vi "Auto Intake Mode.vi"(7 "Intake Current Angle":dbl, 10 "Ball Loaded?":bool) -> (1 "Target Height":dbl, 2 "Roller Speed":dbl, 3 "Angle Power":dbl)   [LabVIEW 2015]
uses:
  Common Code/Intake Commands.ctl
  Robot Global Data.vi
  <vilib>/addons/control/pid/pid.llb/PID (DBL).vi
  <vilib>/addons/control/pid/NI_PID_pid.lvlib
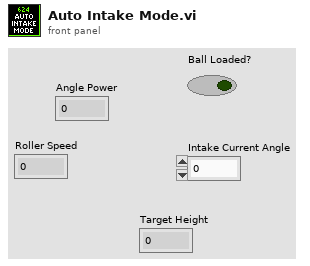
[diagram p1: front panel]
types:
  T1 = typedef "Intake Commands.ctl" = enum16{"Unload", "Load", "Drop low", "Idle"}
  T2 = typedef "Dashboard Control Data.ctl" = cluster{"Encoder Control":T3, "Steer PID output":cluster{"output high":dbl, "output low":dbl}, " Steer PID gains":cluster{"proportional gain (Kc)":dbl, "integral time (Ti, min)":dbl, "derivative time (Td, min)":dbl}, "Drivetrain Settings":T4, "Vision Packet":T5, "Dashboard Drivetrain Command":T6, "Info/Command Cluster":T8, "Ball Vision Packet":T9, "Intake Presets":T11, "Intake Encoder Control":T13, "Climb Presets":T14, "Goal Output Range":cluster{"output high":dbl, "output low":dbl}, "Enabled Systems":T15, "Auton Presets":T16, "Pressure M":dbl, "Pressure B":dbl, "Vision Timeout":dbl, "Auto-Shift":T17, "Catapult Setpoints":T18}
  T3 = typedef "Encoder Control.ctl" = cluster{"Right Tick Constant":dbl, "Left Tick Constant":dbl, "Reset?":bool, "Y Dist":cluster{"PID gains":cluster{"proportional gain (Kc)":dbl, "integral time (Ti, min)":dbl, "derivative time (Td, min)":dbl}}, "Y Stop Thresh":dbl, "Y Stop Speed":dbl}
  T4 = typedef "Drivetrain Settings.ctl" = cluster{"Gyro Tolerance":dbl, "Throttle Ramp (ms)":dbl, "Kv":dbl, "Ka":dbl, "Feed Forward P":dbl, "Feed Forward D":dbl, "Goal Vision PID gains":cluster{"proportional gain (Kc)":dbl, "integral time (Ti, min)":dbl, "derivative time (Td, min)":dbl}, "Goal Detection Window":dbl, "Creep Rate":dbl, "Vision Throttle Threshold":dbl, "Min Turn Output":dbl, "Left Batter Angle":dbl, "Right Batter Angle":dbl}
  T5 = typedef "Goal Vision Packet.ctl" = cluster{"Distance":dbl, "Center X":dbl, "Center Y":dbl, "Found Target?":bool, "Robot Center":dbl, "Angle":dbl}
  T6 = typedef "Dashboard Drivetrain Command.ctl" = cluster{"Drivetrain Vision":T7}
  T7 = typedef "Drivetrain Vision.ctl" = cluster{"Goal Window":dbl, "Ball Window":dbl}
  T8 = typedef "Ball Tracking Command Cluster.ctl" = cluster{"Distance to Ball":dbl, "Desired Angle":dbl, "Command":enum16{"Turn to Ball", "Turn to Angle", "Get Distance"}, "Pixels from Center":dbl}
  T9 = typedef "Ball Vision Packet.ctl" = cluster{"Ball Detected?":bool, "Distance to Ball":dbl, "Desired Angle":dbl, "Pixels from Center":dbl, "Tracking mode":T10}
  T10 = typedef "Tracking Mode.ctl" = enum16{"Turn to Ball", "Turn to Angle"}
  T11 = typedef "Intake Presets.ctl" = cluster{"Intake Speed":dbl, "Outake Speed":dbl, "Angle Speed":dbl, "Angle Tolerance":dbl, "Encoder Scale":dbl, "Load Height":dbl, "Output Range":T12, "MaxCurrent":dbl, "Idle Height":dbl, "Max Height":dbl, "Reset Encoders?":bool, "PID gains":cluster{"proportional gain (Kc)":dbl, "integral time (Ti, min)":dbl, "derivative time (Td, min)":dbl}, "Drop Low Height ":dbl, "Rotation Power Max/Min":dbl}
  T12 = typedef "Drivetrain Output Range.ctl" = cluster{"output high":dbl, "output low":dbl}
  T13 = typedef "IntakeEcoderControl.ctl" = cluster{"Arm Tick Constant":dbl, "Reset?":bool, "Y Dist":cluster{"PID gains":cluster{"proportional gain (Kc)":dbl, "integral time (Ti, min)":dbl, "derivative time (Td, min)":dbl}}, "Y Stop Thresh":dbl, "Y Stop Speed":dbl}
  T14 = typedef "Climb Presets.ctl" = cluster{"Pull Power":dbl, "Extend Power":dbl}
  T15 = typedef "Enabled Systems.ctl" = cluster{"Shoot":bool, "Intake":bool, "DT":bool, "Gyro":bool, "100ms":bool, "US":bool}
  T16 = typedef "Autonomous Presets.ctl" = cluster{"Pitch Limit":dbl, "Roll Limit":dbl, "Start Position":dbl, "Cross Position":dbl}
  T17 = typedef "Auto Shift Cluster.ctl" = cluster{"Delay":dbl, "Speed Thresh":dbl, "Upshift Accel":dbl, "Upshift Throttle":dbl, "Upshift Throttle Accel":dbl, "Downshift Throttle":dbl, "Downshift Throttle Accel":dbl, "Pressure Threshold":dbl}
  T18 = typedef "Catapult Presets.ctl" = cluster{"Intake Danger Height":dbl, "Ball Security Delay ":dbl, "High PSI Minimum":dbl, "Shot Finish Delay":dbl, "Low PSI Minimum":dbl, "Idle Ball Security Wait ":dbl}
  T19 = typedef "Intake Commands Cluster.ctl" = cluster{"Intake Commands":T1, "Intake Mode":T20, "Override IR":bool}
  T20 = typedef "Intake Mode.ctl" = enum16{"Manual", "Safe", "Auto"}
  T21 = cluster{"proportional gain (Kc)":dbl, "integral time (Ti, min)":dbl, "derivative time (Td, min)":dbl}
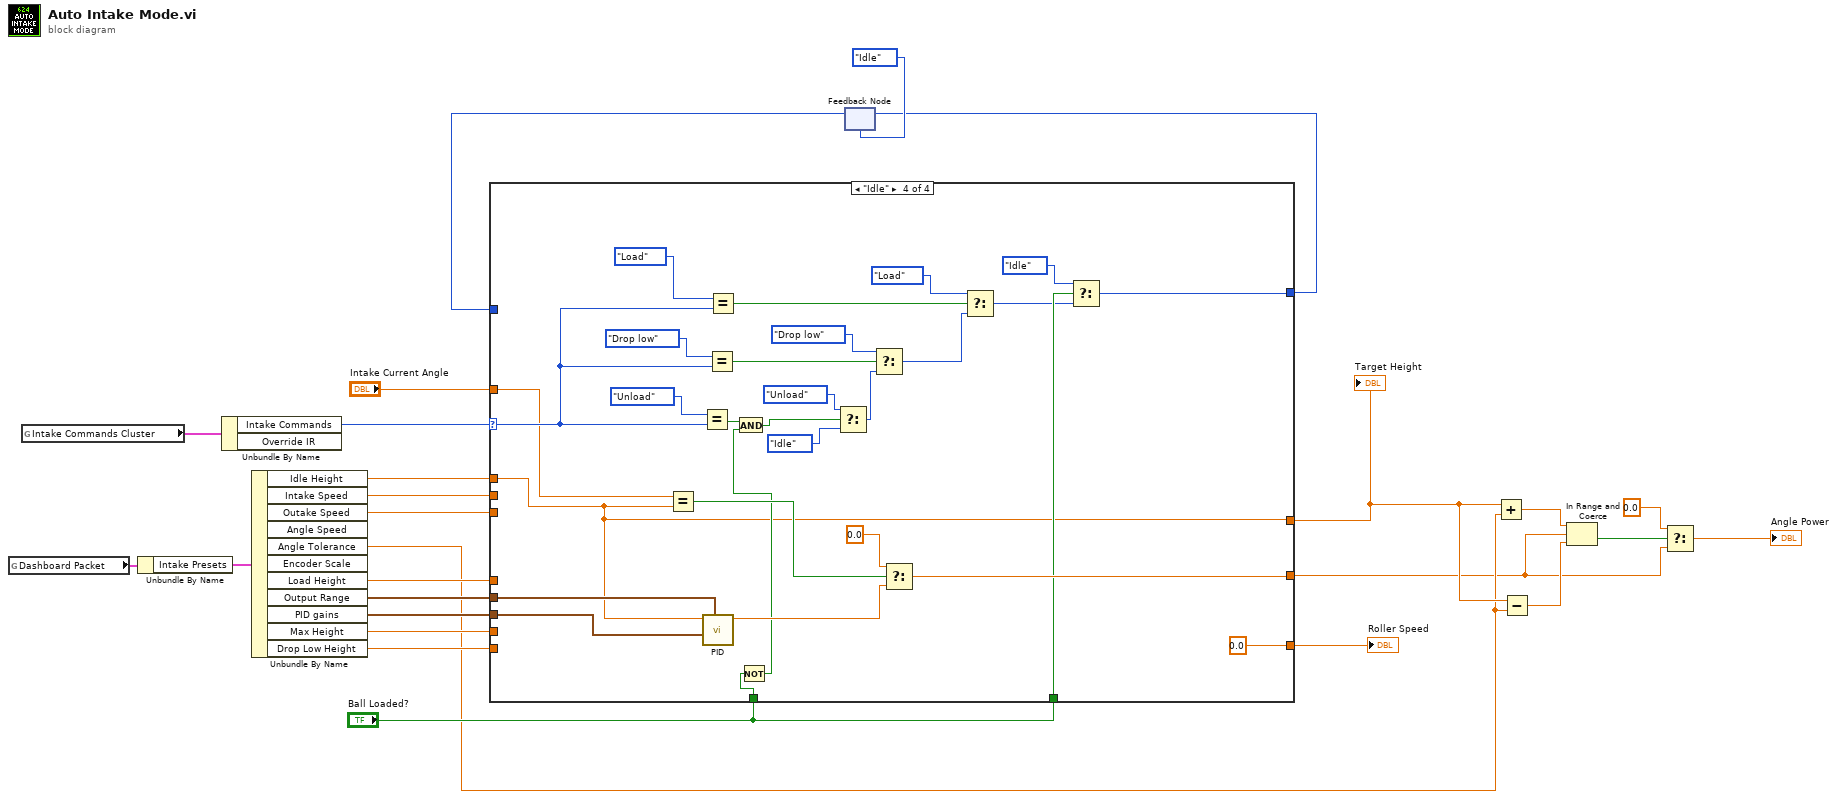
[diagram p0: block diagram]
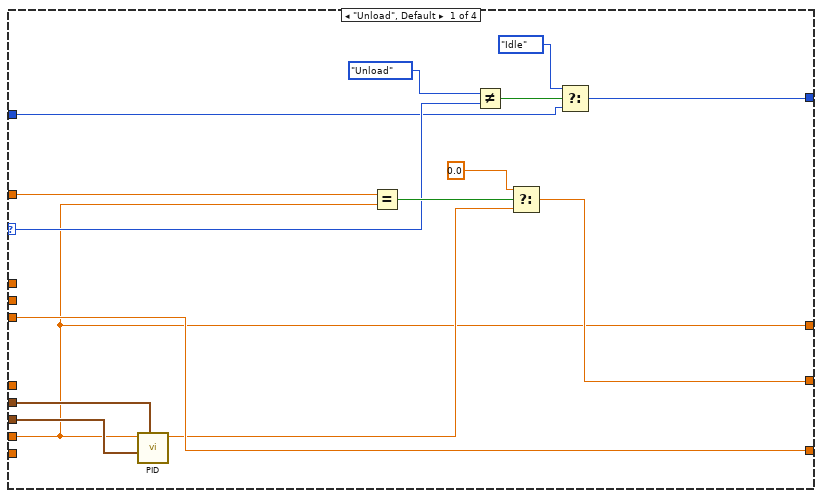
[diagram p2: hidden frame]
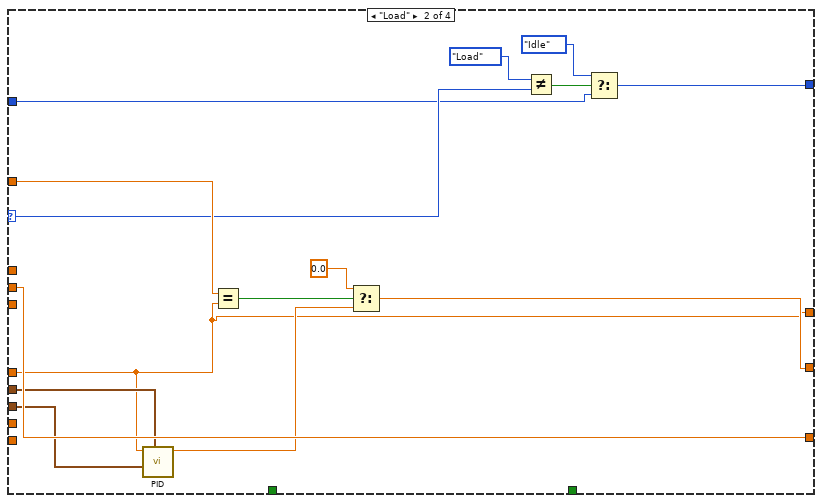
[diagram p3: hidden frame]
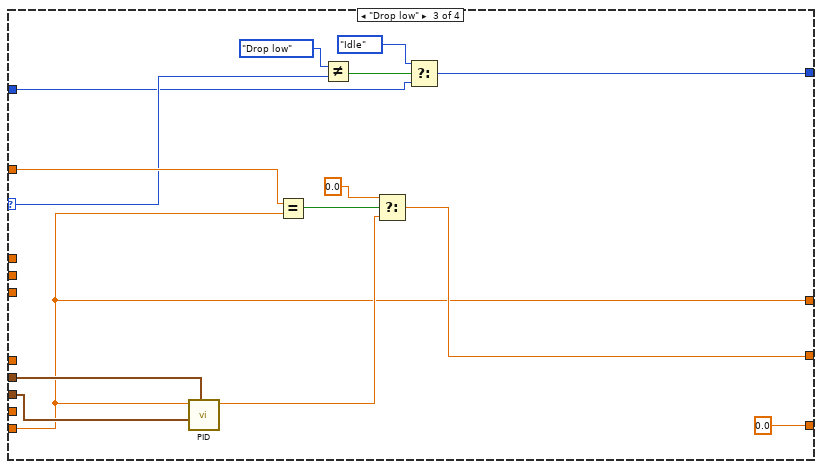
[diagram p4: hidden frame]
diagram:
  n1 = global read "Robot Global Data.vi" "Dashboard Packet"() -> (w24:T2)
  n2 = global read "Robot Global Data.vi" "Intake Commands Cluster"() -> (w26:T19)
  n3 = Unbundle By Name(w24) -> ("Intake Presets"=w23:T11)
  n4 = Unbundle By Name(w26) -> ("Intake Commands"=w25:T1)  [unwired: 1 out]
  n5 = Unbundle By Name(w23) -> ("Idle Height"=w15:dbl, "Intake Speed"=w11:dbl, "Outake Speed"=w14:dbl, "Angle Tolerance"=w3:dbl, "Load Height"=w12:dbl, "Output Range"=w18:T12, "PID gains"=w17:T21, "Max Height"=w13:dbl, "Drop Low Height"=w10:dbl)  [unwired: 2 out]
  n6 = feedback #1(Intake_Commands."Idle" ("Intake Commands")) -> (w21:T1)
  n7 = case shown="\"Idle\"" w25 {
    selector: w25 -> [w33 w48 w63 w91]
    tunnel: w21 -> [w28 w44 w58 _]
    tunnel: [w29 w43 w59 w79] -> w20
    tunnel: [w41 w54 0.0 0.0] -> w19
    tunnel: w18 -> [w37 w53 w68 w87]
    tunnel: w17 -> [w36 w52 w67 w86]
    tunnel: "Intake Current Angle" -> [w40 w56 w71 w82]
    tunnel: w15 -> [_ _ _ w72]
    tunnel: [w34 w49 w65 w84] -> w1
    tunnel: w14 -> [w41 _ _ _]
    tunnel: w13 -> [w27 _ _ _]
    tunnel: w12 -> [_ w42 _ _]
    tunnel: w11 -> [_ w54 _ _]
    tunnel: w10 -> [_ _ w57 _]
    tunnel: "Ball Loaded?" -> [_ _ _ w80]
    tunnel: "Ball Loaded?" -> [_ _ _ w75]
    tunnel: [w27 w42 w57 w72] -> w4
    frame "Unload", Default {
      n8 = call-poly <vilib>:"PID.vi"("output range"=w37, "PID gains"=w36, "setpoint"=w27) -> ("output"=w35:dbl)  [unwired: 7 in, 1 out]
      n9 = Equal?(x=w40, y=w27) -> (x = y?=w39:bool)
      n10 = Not Equal?(x=Intake_Commands."Unload" ("Intake Commands"), y=w33) -> (x != y?=w31:bool)
      n11 = Select(t=0.0, s=w39, f=w35) -> (s? t:f=w34:dbl)
      n12 = Select(t=Intake_Commands."Idle" ("Intake Commands"), s=w31, f=w28) -> (s? t:f=w29:T1)
    }
    frame "Load" {
      n13 = call-poly <vilib>:"PID.vi"("output range"=w53, "PID gains"=w52, "setpoint"=w42) -> ("output"=w51:dbl)  [unwired: 7 in, 1 out]
      n14 = Equal?(x=w56, y=w42) -> (x = y?=w55:bool)
      n15 = Select(t=0.0, s=w55, f=w51) -> (s? t:f=w49:dbl)
      n16 = Not Equal?(x=Intake_Commands."Load" ("Intake Commands"), y=w48) -> (x != y?=w46:bool)
      n17 = Select(t=Intake_Commands."Idle" ("Intake Commands"), s=w46, f=w44) -> (s? t:f=w43:T1)
    }
    frame "Drop low" {
      n18 = call-poly <vilib>:"PID.vi"("output range"=w68, "PID gains"=w67, "setpoint"=w57) -> ("output"=w66:dbl)  [unwired: 7 in, 1 out]
      n19 = Equal?(x=w71, y=w57) -> (x = y?=w70:bool)
      n20 = Not Equal?(x=Intake_Commands."Drop low" ("Intake Commands"), y=w63) -> (x != y?=w61:bool)
      n21 = Select(t=0.0, s=w70, f=w66) -> (s? t:f=w65:dbl)
      n22 = Select(t=Intake_Commands."Idle" ("Intake Commands"), s=w61, f=w58) -> (s? t:f=w59:T1)
    }
    frame "Idle" {
      n23 = Equal?(x=w82, y=w72) -> (x = y?=w85:bool)
      n24 = Equal?(x=Intake_Commands."Unload" ("Intake Commands"), y=w91) -> (x = y?=w76:bool)
      n25 = call-poly <vilib>:"PID.vi"("output range"=w87, "PID gains"=w86, "setpoint"=w72) -> ("output"=w83:dbl)  [unwired: 7 in, 1 out]
      n26 = Equal?(x=Intake_Commands."Drop low" ("Intake Commands"), y=w91) -> (x = y?=w96:bool)
      n27 = Equal?(x=Intake_Commands."Load" ("Intake Commands"), y=w91) -> (x = y?=w99:bool)
      n28 = Not(x=w75) -> (.not. x?=w74:bool)
      n29 = And(x=w76, y=w74) -> (x .and. y?=w73:bool)
      n30 = Select(t=Intake_Commands."Unload" ("Intake Commands"), s=w73, f=Intake_Commands."Idle" ("Intake Commands")) -> (s? t:f=w93:T1)
      n31 = Select(t=Intake_Commands."Drop low" ("Intake Commands"), s=w96, f=w93) -> (s? t:f=w97:T1)
      n32 = Select(t=0.0, s=w85, f=w83) -> (s? t:f=w84:dbl)
      n33 = Select(t=Intake_Commands."Load" ("Intake Commands"), s=w99, f=w97) -> (s? t:f=w78:T1)
      n34 = Select(t=Intake_Commands."Idle" ("Intake Commands"), s=w80, f=w78) -> (s? t:f=w79:T1)
    }
  }
  "Roller Speed" <- w19
  "Target Height" <- w4
  n35 = feedback-in #1(w20) -> ()
  n36 = Add(x=w4, y=w3) -> (x+y=w5:dbl)
  n37 = Subtract(x=w4, y=w3) -> (x-y=w2:dbl)
  n38 = In Range and Coerce(upper limit=w5, x=w1, lower limit=w2) -> (In Range?=w6:bool)  [unwired: 1 out]
  n39 = Select(t=0.0, s=w6, f=w1) -> (s? t:f=→"Angle Power":dbl)
